vi "Send Flags.vi"(8 "error in (no error)":errorcluster, 10 "Flags":T1, 11 "Rover in":refnum<class "Rover.lvclass">) -> (0 "error out":errorcluster, 3 "Rover out":refnum<class "Rover.lvclass">)   [LabVIEW 2020, in "Rover.lvlib" / "Rover.lvclass"]
uses:
  Rover.lvclass
  Flags.ctl
  I2C Register.ctl
  Rover.lvclass/Rover.ctl
  <vilib>/MakerHub/LINX/Private/Local IO/LinxI2cWrite.vi
  <vilib>/MakerHub/LINX/Public/Utilities/Check Channel.vi
  <vilib>/MakerHub/LINX/Private/Local IO/Handle Errors.vi
  <vilib>/MakerHub/LINX/Private/Utilties/Generate Error.vi
  <vilib>/MakerHub/LINX/LMH-LINX.lvlib
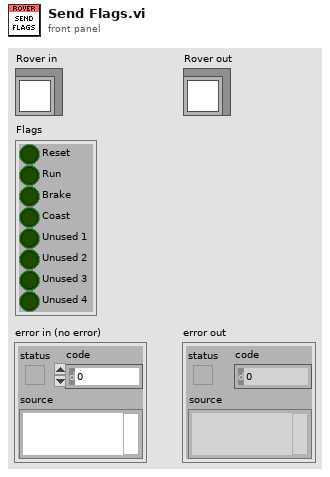
[diagram p1: front panel]
types:
  T1 = typedef "Rover.lvlib/Rover.lvclass/Flags.ctl" = cluster{"Reset":bool, "Run":bool, "Brake":bool, "Coast":bool, "Unused 1":bool, "Unused 2":bool, "Unused 3":bool, "Unused 4":bool}
  T2 = typedef "Rover.lvlib/Rover.lvclass/I2C Register.ctl" = enum8{"encA", "encB", "ticksPerUnit", "width", "flags", "velP", "velI", "velD", "velMin", "velMax", "poseX", "poseY", "poseA", "cmdDrive", "cmdTurn", "velocity", "turn", "velL", "velR", "run", "outL", "outR", "outDeadband"}
  T3 = typedef "LMH-LINX.lvlib/LINX Ref.ctl" = cluster{"IO":T4, "Interface":T5, "LINX Device Config":T6}
  T4 = typedef "LMH-LINX.lvlib/Platform.ctl" = enum16{"Remote", "Local"}
  T5 = typedef "LMH-LINX.lvlib/Interface.ctl" = enum16{"Serial", "TCP"}
  T6 = typedef "LMH-LINX.lvlib/Device.lvlib/LINX Device Config.ctl" = cluster{"Interface":T5, "COM Port":refnum<visa-resource-name>, "TCP Configuration":T7, "Device Family":u8, "Device ID":u8, "Device Name":string, "TCP Ref":refnum<k5>, "Channels":T8}
  T7 = typedef "LMH-LINX.lvlib/Device.lvlib/TCP Config.ctl" = cluster{"IP Address":string, "Port":u16}
  T8 = typedef "LMH-LINX.lvlib/Channels.ctl" = cluster{"DI":u8[], "DO":u8[], "AI":u8[], "AO":u8[], "PWM":u8[], "QE":u8[], "UART":u8[], "I2C 2":u8[], "SPI":u8[], "CAN":u8[], "Servo":u8[], "AI Ref (V)":dbl, "AI Resolution (Bits)":u8, "AO Ref (V)":dbl, "AO Resolution (Bits)":u8}
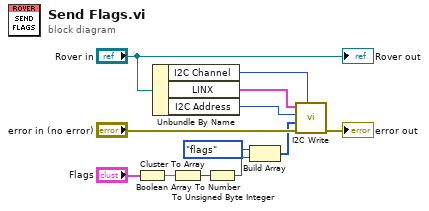
[diagram p0: block diagram]
diagram:
  n1 = Cluster To Array(cluster="Flags") -> (array=w11:bool[])
  n2 = Unbundle By Name("Rover in") -> ("I2C Channel"=w7:u8, "LINX"=w6:T3, "I2C Address"=w5:u8)
  n3 = Boolean Array To Number(Boolean array=w11) -> (number=w10:u32)
  n4 = To Unsigned Byte Integer(number=w10) -> (unsigned 8bit integer=w4:u8)
  n5 = Build Array(I2C_Register."flags" ("I2C Register"), w4) -> (w2:u8[])
  n6 = call <vilib>:"I2C Write.vi"("I2C Channel"=w7, "Error In"="error in (no error)", "Data"=w2, "I2C Slave Address (0)"=w5, "LINX Resource"=w6) -> ("Error Out"=→"error out":errorcluster)  [unwired: 5 in, 1 out]
  "Rover out" <- "Rover in"
